vi "PicoScope4000aProbeSettings.vi"(0 "handle in":i16, 1 "Device Info":T3={"Driver Version"="", "USB Version"="", "Hardware"="", "Variant"="", "Batch and Serial"="", "Cal Date"="", "Kernel Version"="", "Digital HW Version"="", "Analogue HW Version"="", "Firmware 1"="", "Firmware 2"="", "Num. channels"=4}, 4 "Probe Input Array":T5(array[cluster])=[{"probeNumber"=0, FALSE, "channel"=-1, "enabled"=0, "probeName"=0, "requiresPower"=0, "isPowered"=0, "probeOff"=0, "rangeFirst"=0, "rangeLast"=0, "rangeCurrent"=0, "couplingFirst"=0, "couplingLast"=0, "couplingCurrent"=0, "filterFlags"=0, "filterCurrent"=0, "defaultFilter"=0}, {"probeNumber"=0, FALSE, "channel"=-1, "enabled"=0, "probeName"=0, "requiresPower"=0, "isPowered"=0, "probeOff"=0, "rangeFirst"=0, "rangeLast"=0, "rangeCurrent"=0, "couplingFirst"=0, "couplingLast"=0, "couplingCurrent"=0, "filterFlags"=0, "filterCurrent"=0, "defaultFilter"=0}, {"probeNumber"=0, FALSE, "channel"=-1, "enabled"=0, "probeName"=0, "requiresPower"=0, "isPowered"=0, "probeOff"=0, "rangeFirst"=0, "rangeLast"=0, "rangeCurrent"=0, "couplingFirst"=0, "couplingLast"=0, "couplingCurrent"=0, "filterFlags"=0, "filterCurrent"=0, "defaultFilter"=0}, {"probeNumber"=0, FALSE, "channel"=-1, "enabled"=0, "probeName"=0, "requiresPower"=0, "isPowered"=0, "probeOff"=0, "rangeFirst"=0, "rangeLast"=0, "rangeCurrent"=0, "couplingFirst"=0, "couplingLast"=0, "couplingCurrent"=0, "filterFlags"=0, "filterCurrent"=0, "defaultFilter"=0}], 5 "error in (no error)":errorcluster, 6 "Channel A Settings":T4={"Enabled"=FALSE, "Coupling"=1, "Range"=0, "Analogue Offset"=0.0, "Bandwidth Limit"=0} {"Range" items=["10mV"=0, "20mV"=1, "50mV"=2, "100mV"=3, "200mV"=4, "500mV"=5, "1V"=6, "2V"=7, "5V"=8, "10V"=9, "20V"=10, "50V"=11, "100V"=12, "200V"=13, "1KV_2_5V"=6003, "1KV_5V"=6004, "1KV_12_5V"=6005, "1KV_25V"=6006, "1KV_50V"=6007, "1KV_125V"=6008, "1KV_250V"=6009, "1KV_500V"=6010, "1KV_1000V"=6011, "CURRENT_CLAMP_200A_2kA_1A"=4000, "CURRENT_CLAMP_200A_2kA_2A"=4001, "CURRENT_CLAMP_200A_2kA_5A"=4002, "CURRENT_CLAMP_200A_2kA_10A"=4003, "CURRENT_CLAMP_200A_2kA_20A"=4004, "CURRENT_CLAMP_200A_2kA_50A"=4005, "CURRENT_CLAMP_200A_2kA_100A"=4006, "CURRENT_CLAMP_200A_2kA_200A"=4007, "CURRENT_CLAMP_200A_2kA_500A"=4008, "CURRENT_CLAMP_200A_2kA_1000A"=4009, "CURRENT_CLAMP_200A_2kA_2000A"=4010, "CURRENT_CLAMP_40A_100mA"=5000, "CURRENT_CLAMP_40A_200mA"=5001, "CURRENT_CLAMP_40A_500mA"=5002, "CURRENT_CLAMP_40A_1A"=5003, "CURRENT_CLAMP_40A_2A"=5004, "CURRENT_CLAMP_40A_5A"=5005, "CURRENT_CLAMP_40A_10A"=5006, "CURRENT_CLAMP_40A_20A"=5007, "CURRENT_CLAMP_40A_40A"=5008, "CURRENT_CLAMP_2000ARMS_10A"=6500, "CURRENT_CLAMP_2000ARMS_20A"=6501, "CURRENT_CLAMP_2000ARMS_50A"=6502, "CURRENT_CLAMP_2000ARMS_100A"=6503, "CURRENT_CLAMP_2000ARMS_200A"=6504, "CURRENT_CLAMP_2000ARMS_500A"=6505, "CURRENT_CLAMP_2000ARMS_1000A"=6506, "CURRENT_CLAMP_2000ARMS_2000A"=6507, "CURRENT_CLAMP_2000ARMS_5000A"=6508, "x10_Probe_100mV"=32, "x10_Probe_200mV"=33, "x10_Probe_500mV"=34, "x10_Probe_1V"=35, "x10_Probe_2V"=36, "x10_Probe_5V"=37, "x10_Probe_10V"=38, "x10_Probe_20V"=39, "x10_Probe_50V"=40, "x10_Probe_100V"=41, "x10_Probe_200V"=42, "x10_Probe_500V"=43, "CURRENT_CLAMP_60A_2A"=10500, "CURRENT_CLAMP_60A_5A"=10501, "CURRENT_CLAMP_60A_10A"=10502, "CURRENT_CLAMP_60A_20A"=10503, "CURRENT_CLAMP_60A_50A"=10504, "CURRENT_CLAMP_60A_60A"=10505, "CURRENT_CLAMP_60A_V2_0_5A"=10600, "CURRENT_CLAMP_60A_V2_1A"=10601, "CURRENT_CLAMP_60A_V2_2A"=10602, "CURRENT_CLAMP_60A_V2_5A"=10603, "CURRENT_CLAMP_60A_V2_10A"=10604, "CURRENT_CLAMP_60A_V2_20A"=10605, "CURRENT_CLAMP_60A_V2_50A"=10606, "CURRENT_CLAMP_60A_V2_60A"=10607, "RESISTANCE_LEAD_NEG5_TO_20OHM"=7000, "RESISTANCE_LEAD_NEG50_TO_200OHM"=7001, "RESISTANCE_LEAD_NEG500_TO_2KOHM"=7002, "RESISTANCE_LEAD_NEG5K_TO_20KOHM"=7003, "RESISTANCE_LEAD_NEG50K_TO_LEAD_200KOHM"=7004, "RESISTANCE_LEAD_NEG500K_TO_LEAD_2MOHM"=7005, "RESISTANCE_LEAD_DIODE_TEST"=7006, "HT_NEG3_TO_5KV"=8950, "HT_NEG3_TO_10KV"=8951, "HT_NEG5_TO_20KV"=8952, "HT_NEG5_TO_50KV"=8953, "HT_NEG5_TO_100KV"=8954, "HT_NEG3_TO_5KV_INVERTED"=8955, "HT_NEG3_TO_10KV_INVERTED"=8956, "HT_NEG5_TO_20KV_INVERTED"=8957, "HT_NEG5_TO_50KV_INVERTED"=8958, "HT_NEG5_TO_100KV_INVERTED"=8959, "TEMPERATURE_NEG50_TO_150DEGC"=9000, "PRESSURE_SENSOR_-100k-150k_PASCALS"=9100, "PRESSURE_SENSOR_-100k_TO_400k_PASCALS"=9101, "PRESSURE_SENSOR_-200k_TO_800k_PASCALS"=9102, "PRESSURE_SENSOR_-400k_TO_1600k_PASCALS"=9103, "PRESSURE_SENSOR_-400k_TO_3400k_PASCALS"=9104, "PRESSURE_SENSOR_-150k_TO_1350k_PASCALS"=9105, "PICO_CONNECT_PROBE_OFF"=1024]; "Bandwidth Limit" items=["Full", "20kHz", "100kHz", "1MHz"]; "Coupling" items=["AC", "DC"]}, 8 "Channel B Settings":T4={"Enabled"=FALSE, "Coupling"=1, "Range"=0, "Analogue Offset"=0.0, "Bandwidth Limit"=0} {"Range" items=["10mV"=0, "20mV"=1, "50mV"=2, "100mV"=3, "200mV"=4, "500mV"=5, "1V"=6, "2V"=7, "5V"=8, "10V"=9, "20V"=10, "50V"=11, "100V"=12, "200V"=13, "1KV_2_5V"=6003, "1KV_5V"=6004, "1KV_12_5V"=6005, "1KV_25V"=6006, "1KV_50V"=6007, "1KV_125V"=6008, "1KV_250V"=6009, "1KV_500V"=6010, "1KV_1000V"=6011, "CURRENT_CLAMP_200A_2kA_1A"=4000, "CURRENT_CLAMP_200A_2kA_2A"=4001, "CURRENT_CLAMP_200A_2kA_5A"=4002, "CURRENT_CLAMP_200A_2kA_10A"=4003, "CURRENT_CLAMP_200A_2kA_20A"=4004, "CURRENT_CLAMP_200A_2kA_50A"=4005, "CURRENT_CLAMP_200A_2kA_100A"=4006, "CURRENT_CLAMP_200A_2kA_200A"=4007, "CURRENT_CLAMP_200A_2kA_500A"=4008, "CURRENT_CLAMP_200A_2kA_1000A"=4009, "CURRENT_CLAMP_200A_2kA_2000A"=4010, "CURRENT_CLAMP_40A_100mA"=5000, "CURRENT_CLAMP_40A_200mA"=5001, "CURRENT_CLAMP_40A_500mA"=5002, "CURRENT_CLAMP_40A_1A"=5003, "CURRENT_CLAMP_40A_2A"=5004, "CURRENT_CLAMP_40A_5A"=5005, "CURRENT_CLAMP_40A_10A"=5006, "CURRENT_CLAMP_40A_20A"=5007, "CURRENT_CLAMP_40A_40A"=5008, "CURRENT_CLAMP_2000ARMS_10A"=6500, "CURRENT_CLAMP_2000ARMS_20A"=6501, "CURRENT_CLAMP_2000ARMS_50A"=6502, "CURRENT_CLAMP_2000ARMS_100A"=6503, "CURRENT_CLAMP_2000ARMS_200A"=6504, "CURRENT_CLAMP_2000ARMS_500A"=6505, "CURRENT_CLAMP_2000ARMS_1000A"=6506, "CURRENT_CLAMP_2000ARMS_2000A"=6507, "CURRENT_CLAMP_2000ARMS_5000A"=6508, "x10_Probe_100mV"=32, "x10_Probe_200mV"=33, "x10_Probe_500mV"=34, "x10_Probe_1V"=35, "x10_Probe_2V"=36, "x10_Probe_5V"=37, "x10_Probe_10V"=38, "x10_Probe_20V"=39, "x10_Probe_50V"=40, "x10_Probe_100V"=41, "x10_Probe_200V"=42, "x10_Probe_500V"=43, "CURRENT_CLAMP_60A_2A"=10500, "CURRENT_CLAMP_60A_5A"=10501, "CURRENT_CLAMP_60A_10A"=10502, "CURRENT_CLAMP_60A_20A"=10503, "CURRENT_CLAMP_60A_50A"=10504, "CURRENT_CLAMP_60A_60A"=10505, "CURRENT_CLAMP_60A_V2_0_5A"=10600, "CURRENT_CLAMP_60A_V2_1A"=10601, "CURRENT_CLAMP_60A_V2_2A"=10602, "CURRENT_CLAMP_60A_V2_5A"=10603, "CURRENT_CLAMP_60A_V2_10A"=10604, "CURRENT_CLAMP_60A_V2_20A"=10605, "CURRENT_CLAMP_60A_V2_50A"=10606, "CURRENT_CLAMP_60A_V2_60A"=10607, "RESISTANCE_LEAD_NEG5_TO_20OHM"=7000, "RESISTANCE_LEAD_NEG50_TO_200OHM"=7001, "RESISTANCE_LEAD_NEG500_TO_2KOHM"=7002, "RESISTANCE_LEAD_NEG5K_TO_20KOHM"=7003, "RESISTANCE_LEAD_NEG50K_TO_LEAD_200KOHM"=7004, "RESISTANCE_LEAD_NEG500K_TO_LEAD_2MOHM"=7005, "RESISTANCE_LEAD_DIODE_TEST"=7006, "HT_NEG3_TO_5KV"=8950, "HT_NEG3_TO_10KV"=8951, "HT_NEG5_TO_20KV"=8952, "HT_NEG5_TO_50KV"=8953, "HT_NEG5_TO_100KV"=8954, "HT_NEG3_TO_5KV_INVERTED"=8955, "HT_NEG3_TO_10KV_INVERTED"=8956, "HT_NEG5_TO_20KV_INVERTED"=8957, "HT_NEG5_TO_50KV_INVERTED"=8958, "HT_NEG5_TO_100KV_INVERTED"=8959, "TEMPERATURE_NEG50_TO_150DEGC"=9000, "PRESSURE_SENSOR_-100k-150k_PASCALS"=9100, "PRESSURE_SENSOR_-100k_TO_400k_PASCALS"=9101, "PRESSURE_SENSOR_-200k_TO_800k_PASCALS"=9102, "PRESSURE_SENSOR_-400k_TO_1600k_PASCALS"=9103, "PRESSURE_SENSOR_-400k_TO_3400k_PASCALS"=9104, "PRESSURE_SENSOR_-150k_TO_1350k_PASCALS"=9105, "PICO_CONNECT_PROBE_OFF"=1024]; "Bandwidth Limit" items=["Full", "20kHz", "100kHz", "1MHz"]; "Coupling" items=["AC", "DC"]}, 10 "Channel C Settings":T4={"Enabled"=FALSE, "Coupling"=1, "Range"=0, "Analogue Offset"=0.0, "Bandwidth Limit"=0} {"Range" items=["10mV"=0, "20mV"=1, "50mV"=2, "100mV"=3, "200mV"=4, "500mV"=5, "1V"=6, "2V"=7, "5V"=8, "10V"=9, "20V"=10, "50V"=11, "100V"=12, "200V"=13, "1KV_2_5V"=6003, "1KV_5V"=6004, "1KV_12_5V"=6005, "1KV_25V"=6006, "1KV_50V"=6007, "1KV_125V"=6008, "1KV_250V"=6009, "1KV_500V"=6010, "1KV_1000V"=6011, "CURRENT_CLAMP_200A_2kA_1A"=4000, "CURRENT_CLAMP_200A_2kA_2A"=4001, "CURRENT_CLAMP_200A_2kA_5A"=4002, "CURRENT_CLAMP_200A_2kA_10A"=4003, "CURRENT_CLAMP_200A_2kA_20A"=4004, "CURRENT_CLAMP_200A_2kA_50A"=4005, "CURRENT_CLAMP_200A_2kA_100A"=4006, "CURRENT_CLAMP_200A_2kA_200A"=4007, "CURRENT_CLAMP_200A_2kA_500A"=4008, "CURRENT_CLAMP_200A_2kA_1000A"=4009, "CURRENT_CLAMP_200A_2kA_2000A"=4010, "CURRENT_CLAMP_40A_100mA"=5000, "CURRENT_CLAMP_40A_200mA"=5001, "CURRENT_CLAMP_40A_500mA"=5002, "CURRENT_CLAMP_40A_1A"=5003, "CURRENT_CLAMP_40A_2A"=5004, "CURRENT_CLAMP_40A_5A"=5005, "CURRENT_CLAMP_40A_10A"=5006, "CURRENT_CLAMP_40A_20A"=5007, "CURRENT_CLAMP_40A_40A"=5008, "CURRENT_CLAMP_2000ARMS_10A"=6500, "CURRENT_CLAMP_2000ARMS_20A"=6501, "CURRENT_CLAMP_2000ARMS_50A"=6502, "CURRENT_CLAMP_2000ARMS_100A"=6503, "CURRENT_CLAMP_2000ARMS_200A"=6504, "CURRENT_CLAMP_2000ARMS_500A"=6505, "CURRENT_CLAMP_2000ARMS_1000A"=6506, "CURRENT_CLAMP_2000ARMS_2000A"=6507, "CURRENT_CLAMP_2000ARMS_5000A"=6508, "x10_Probe_100mV"=32, "x10_Probe_200mV"=33, "x10_Probe_500mV"=34, "x10_Probe_1V"=35, "x10_Probe_2V"=36, "x10_Probe_5V"=37, "x10_Probe_10V"=38, "x10_Probe_20V"=39, "x10_Probe_50V"=40, "x10_Probe_100V"=41, "x10_Probe_200V"=42, "x10_Probe_500V"=43, "CURRENT_CLAMP_60A_2A"=10500, "CURRENT_CLAMP_60A_5A"=10501, "CURRENT_CLAMP_60A_10A"=10502, "CURRENT_CLAMP_60A_20A"=10503, "CURRENT_CLAMP_60A_50A"=10504, "CURRENT_CLAMP_60A_60A"=10505, "CURRENT_CLAMP_60A_V2_0_5A"=10600, "CURRENT_CLAMP_60A_V2_1A"=10601, "CURRENT_CLAMP_60A_V2_2A"=10602, "CURRENT_CLAMP_60A_V2_5A"=10603, "CURRENT_CLAMP_60A_V2_10A"=10604, "CURRENT_CLAMP_60A_V2_20A"=10605, "CURRENT_CLAMP_60A_V2_50A"=10606, "CURRENT_CLAMP_60A_V2_60A"=10607, "RESISTANCE_LEAD_NEG5_TO_20OHM"=7000, "RESISTANCE_LEAD_NEG50_TO_200OHM"=7001, "RESISTANCE_LEAD_NEG500_TO_2KOHM"=7002, "RESISTANCE_LEAD_NEG5K_TO_20KOHM"=7003, "RESISTANCE_LEAD_NEG50K_TO_LEAD_200KOHM"=7004, "RESISTANCE_LEAD_NEG500K_TO_LEAD_2MOHM"=7005, "RESISTANCE_LEAD_DIODE_TEST"=7006, "HT_NEG3_TO_5KV"=8950, "HT_NEG3_TO_10KV"=8951, "HT_NEG5_TO_20KV"=8952, "HT_NEG5_TO_50KV"=8953, "HT_NEG5_TO_100KV"=8954, "HT_NEG3_TO_5KV_INVERTED"=8955, "HT_NEG3_TO_10KV_INVERTED"=8956, "HT_NEG5_TO_20KV_INVERTED"=8957, "HT_NEG5_TO_50KV_INVERTED"=8958, "HT_NEG5_TO_100KV_INVERTED"=8959, "TEMPERATURE_NEG50_TO_150DEGC"=9000, "PRESSURE_SENSOR_-100k-150k_PASCALS"=9100, "PRESSURE_SENSOR_-100k_TO_400k_PASCALS"=9101, "PRESSURE_SENSOR_-200k_TO_800k_PASCALS"=9102, "PRESSURE_SENSOR_-400k_TO_1600k_PASCALS"=9103, "PRESSURE_SENSOR_-400k_TO_3400k_PASCALS"=9104, "PRESSURE_SENSOR_-150k_TO_1350k_PASCALS"=9105, "PICO_CONNECT_PROBE_OFF"=1024]; "Bandwidth Limit" items=["Full", "20kHz", "100kHz", "1MHz"]; "Coupling" items=["AC", "DC"]}, 12 "Channel D Settings":T4={"Enabled"=FALSE, "Coupling"=1, "Range"=0, "Analogue Offset"=0.0, "Bandwidth Limit"=0} {"Range" items=["10mV"=0, "20mV"=1, "50mV"=2, "100mV"=3, "200mV"=4, "500mV"=5, "1V"=6, "2V"=7, "5V"=8, "10V"=9, "20V"=10, "50V"=11, "100V"=12, "200V"=13, "1KV_2_5V"=6003, "1KV_5V"=6004, "1KV_12_5V"=6005, "1KV_25V"=6006, "1KV_50V"=6007, "1KV_125V"=6008, "1KV_250V"=6009, "1KV_500V"=6010, "1KV_1000V"=6011, "CURRENT_CLAMP_200A_2kA_1A"=4000, "CURRENT_CLAMP_200A_2kA_2A"=4001, "CURRENT_CLAMP_200A_2kA_5A"=4002, "CURRENT_CLAMP_200A_2kA_10A"=4003, "CURRENT_CLAMP_200A_2kA_20A"=4004, "CURRENT_CLAMP_200A_2kA_50A"=4005, "CURRENT_CLAMP_200A_2kA_100A"=4006, "CURRENT_CLAMP_200A_2kA_200A"=4007, "CURRENT_CLAMP_200A_2kA_500A"=4008, "CURRENT_CLAMP_200A_2kA_1000A"=4009, "CURRENT_CLAMP_200A_2kA_2000A"=4010, "CURRENT_CLAMP_40A_100mA"=5000, "CURRENT_CLAMP_40A_200mA"=5001, "CURRENT_CLAMP_40A_500mA"=5002, "CURRENT_CLAMP_40A_1A"=5003, "CURRENT_CLAMP_40A_2A"=5004, "CURRENT_CLAMP_40A_5A"=5005, "CURRENT_CLAMP_40A_10A"=5006, "CURRENT_CLAMP_40A_20A"=5007, "CURRENT_CLAMP_40A_40A"=5008, "CURRENT_CLAMP_2000ARMS_10A"=6500, "CURRENT_CLAMP_2000ARMS_20A"=6501, "CURRENT_CLAMP_2000ARMS_50A"=6502, "CURRENT_CLAMP_2000ARMS_100A"=6503, "CURRENT_CLAMP_2000ARMS_200A"=6504, "CURRENT_CLAMP_2000ARMS_500A"=6505, "CURRENT_CLAMP_2000ARMS_1000A"=6506, "CURRENT_CLAMP_2000ARMS_2000A"=6507, "CURRENT_CLAMP_2000ARMS_5000A"=6508, "x10_Probe_100mV"=32, "x10_Probe_200mV"=33, "x10_Probe_500mV"=34, "x10_Probe_1V"=35, "x10_Probe_2V"=36, "x10_Probe_5V"=37, "x10_Probe_10V"=38, "x10_Probe_20V"=39, "x10_Probe_50V"=40, "x10_Probe_100V"=41, "x10_Probe_200V"=42, "x10_Probe_500V"=43, "CURRENT_CLAMP_60A_2A"=10500, "CURRENT_CLAMP_60A_5A"=10501, "CURRENT_CLAMP_60A_10A"=10502, "CURRENT_CLAMP_60A_20A"=10503, "CURRENT_CLAMP_60A_50A"=10504, "CURRENT_CLAMP_60A_60A"=10505, "CURRENT_CLAMP_60A_V2_0_5A"=10600, "CURRENT_CLAMP_60A_V2_1A"=10601, "CURRENT_CLAMP_60A_V2_2A"=10602, "CURRENT_CLAMP_60A_V2_5A"=10603, "CURRENT_CLAMP_60A_V2_10A"=10604, "CURRENT_CLAMP_60A_V2_20A"=10605, "CURRENT_CLAMP_60A_V2_50A"=10606, "CURRENT_CLAMP_60A_V2_60A"=10607, "RESISTANCE_LEAD_NEG5_TO_20OHM"=7000, "RESISTANCE_LEAD_NEG50_TO_200OHM"=7001, "RESISTANCE_LEAD_NEG500_TO_2KOHM"=7002, "RESISTANCE_LEAD_NEG5K_TO_20KOHM"=7003, "RESISTANCE_LEAD_NEG50K_TO_LEAD_200KOHM"=7004, "RESISTANCE_LEAD_NEG500K_TO_LEAD_2MOHM"=7005, "RESISTANCE_LEAD_DIODE_TEST"=7006, "HT_NEG3_TO_5KV"=8950, "HT_NEG3_TO_10KV"=8951, "HT_NEG5_TO_20KV"=8952, "HT_NEG5_TO_50KV"=8953, "HT_NEG5_TO_100KV"=8954, "HT_NEG3_TO_5KV_INVERTED"=8955, "HT_NEG3_TO_10KV_INVERTED"=8956, "HT_NEG5_TO_20KV_INVERTED"=8957, "HT_NEG5_TO_50KV_INVERTED"=8958, "HT_NEG5_TO_100KV_INVERTED"=8959, "TEMPERATURE_NEG50_TO_150DEGC"=9000, "PRESSURE_SENSOR_-100k-150k_PASCALS"=9100, "PRESSURE_SENSOR_-100k_TO_400k_PASCALS"=9101, "PRESSURE_SENSOR_-200k_TO_800k_PASCALS"=9102, "PRESSURE_SENSOR_-400k_TO_1600k_PASCALS"=9103, "PRESSURE_SENSOR_-400k_TO_3400k_PASCALS"=9104, "PRESSURE_SENSOR_-150k_TO_1350k_PASCALS"=9105, "PICO_CONNECT_PROBE_OFF"=1024]; "Bandwidth Limit" items=["Full", "20kHz", "100kHz", "1MHz"]; "Coupling" items=["AC", "DC"]}) -> (7 "ChA":T2={"Probe Info"={"Ch Min Limit"=0.0, "Ch Max Limit"=0.0, "Probe Name"=0}, "Channel A Settings "={"Enabled"=FALSE, "Coupling"=1, "Range"=0, "Analogue Offset"=0.0, "Bandwidth Limit"=0}} {"Channel A Settings"."Bandwidth Limit" items=["Full", "20kHz", "100kHz", "1MHz"]; "Channel A Settings"."Range" items=["10 mV", "20 mV", "50 mV", "100 mV", "200 mV", "500 mV", "1 V", "2 V", "5 V", "10 V", "20 V", "50 V ", "100 V"]; "Channel A Settings"."Coupling" items=["AC", "DC"]}, 9 "ChB":T2={"Probe Info"={"Ch Min Limit"=0.0, "Ch Max Limit"=0.0, "Probe Name"=0}, "Channel A Settings "={"Enabled"=FALSE, "Coupling"=1, "Range"=0, "Analogue Offset"=0.0, "Bandwidth Limit"=0}} {"Channel A Settings"."Bandwidth Limit" items=["Full", "20kHz", "100kHz", "1MHz"]; "Channel A Settings"."Range" items=["10 mV", "20 mV", "50 mV", "100 mV", "200 mV", "500 mV", "1 V", "2 V", "5 V", "10 V", "20 V", "50 V ", "100 V"]; "Channel A Settings"."Coupling" items=["AC", "DC"]}, 11 "ChC":T2={"Probe Info"={"Ch Min Limit"=0.0, "Ch Max Limit"=0.0, "Probe Name"=0}, "Channel A Settings "={"Enabled"=FALSE, "Coupling"=1, "Range"=0, "Analogue Offset"=0.0, "Bandwidth Limit"=0}} {"Channel A Settings"."Bandwidth Limit" items=["Full", "20kHz", "100kHz", "1MHz"]; "Channel A Settings"."Range" items=["10 mV", "20 mV", "50 mV", "100 mV", "200 mV", "500 mV", "1 V", "2 V", "5 V", "10 V", "20 V", "50 V ", "100 V"]; "Channel A Settings"."Coupling" items=["AC", "DC"]}, 13 "ChD":T2={"Probe Info"={"Ch Min Limit"=0.0, "Ch Max Limit"=0.0, "Probe Name"=0}, "Channel A Settings "={"Enabled"=FALSE, "Coupling"=1, "Range"=0, "Analogue Offset"=0.0, "Bandwidth Limit"=0}} {"Channel A Settings"."Bandwidth Limit" items=["Full", "20kHz", "100kHz", "1MHz"]; "Channel A Settings"."Range" items=["10 mV", "20 mV", "50 mV", "100 mV", "200 mV", "500 mV", "1 V", "2 V", "5 V", "10 V", "20 V", "50 V ", "100 V"]; "Channel A Settings"."Coupling" items=["AC", "DC"]}, 14 "handle out":i16, 19 "error out":errorcluster)   [LabVIEW 2010]
uses:
  PicoScope4000aAnalogChannelSettings.ctl
  PicoScope4000aAnalogChannelSettings_PicoConnect.ctl
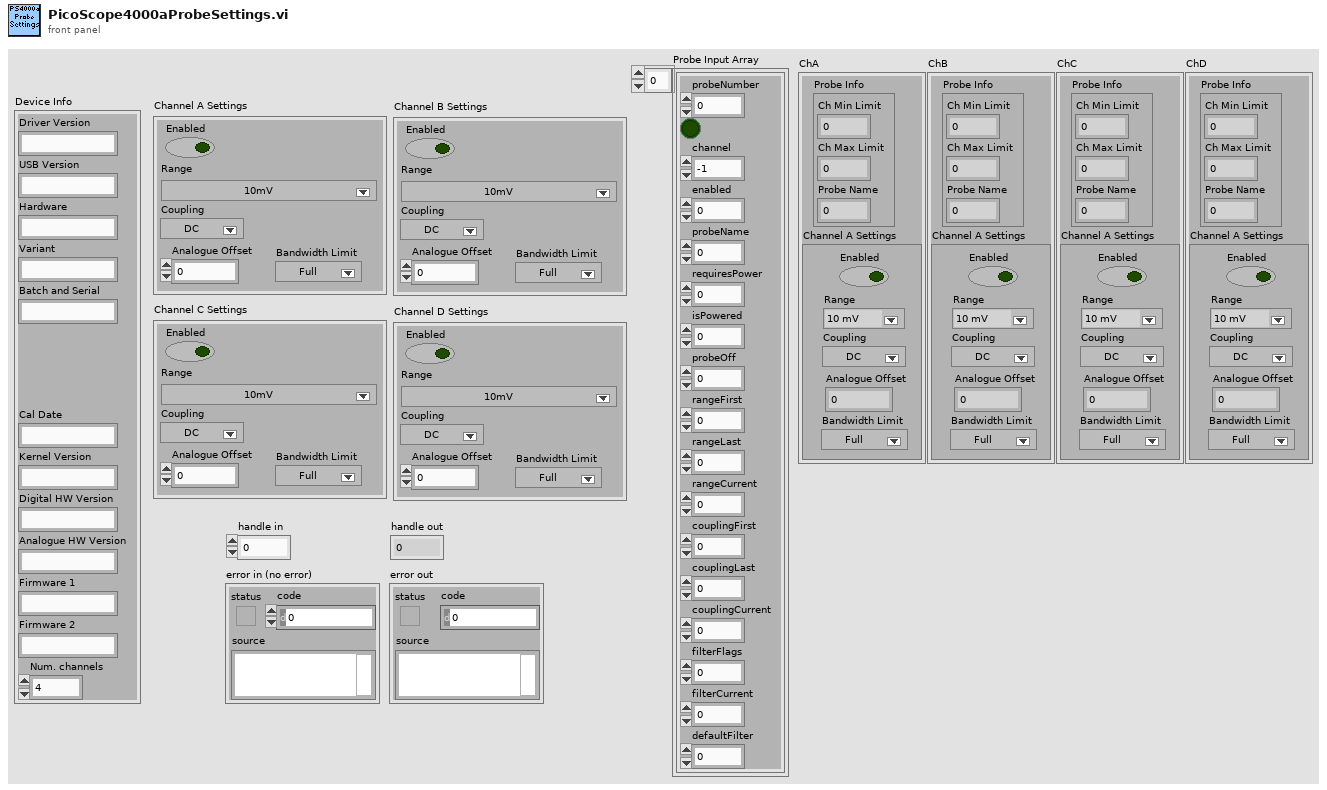
[diagram p1: front panel]
types:
  T1 = typedef "PicoScope4000aAnalogChannelSettings.ctl" = cluster{"Enabled":bool, "Coupling":i16, "Range":u32, "Analogue Offset":sgl, "Bandwidth Limit":u32}
  T2 = cluster{"Probe Info":cluster{"Ch Min Limit":dbl, "Ch Max Limit":dbl, "Probe Name":i32}, "Channel A Settings ":T1}
  T3 = cluster{"Driver Version":string, "USB Version":string, "Hardware":string, "Variant":string, "Batch and Serial":string, "Cal Date":string, "Kernel Version":string, "Digital HW Version":string, "Analogue HW Version":string, "Firmware 1":string, "Firmware 2":string, "Num. channels":i16}
  T4 = typedef "PicoScope4000aAnalogChannelSettings_PicoConnect.ctl" = cluster{"Enabled":bool, "Coupling":i16, "Range":u32, "Analogue Offset":sgl, "Bandwidth Limit":u32}
  T5 = cluster{"probeNumber":i32, bool, "channel":i32, "enabled":i16, "probeName":i32, "requiresPower":i8, "isPowered":i8, "probeOff":i32, "rangeFirst":i32, "rangeLast":i32, "rangeCurrent":i32, "couplingFirst":i32, "couplingLast":i32, "couplingCurrent":i32, "filterFlags":i32, "filterCurrent":i32, "defaultFilter":i32}[]
  T6 = cluster{"Ch Min Limit":dbl, "Ch Max Limit":dbl, "Probe Name":i32}
  T7 = cluster{"probeNumber":i32, bool, "channel":i32, "enabled":i16, "probeName":i32, "requiresPower":i8, "isPowered":i8, "probeOff":i32, "rangeFirst":i32, "rangeLast":i32, "rangeCurrent":i32, "couplingFirst":i32, "couplingLast":i32, "couplingCurrent":i32, "filterFlags":i32, "filterCurrent":i32, "defaultFilter":i32}
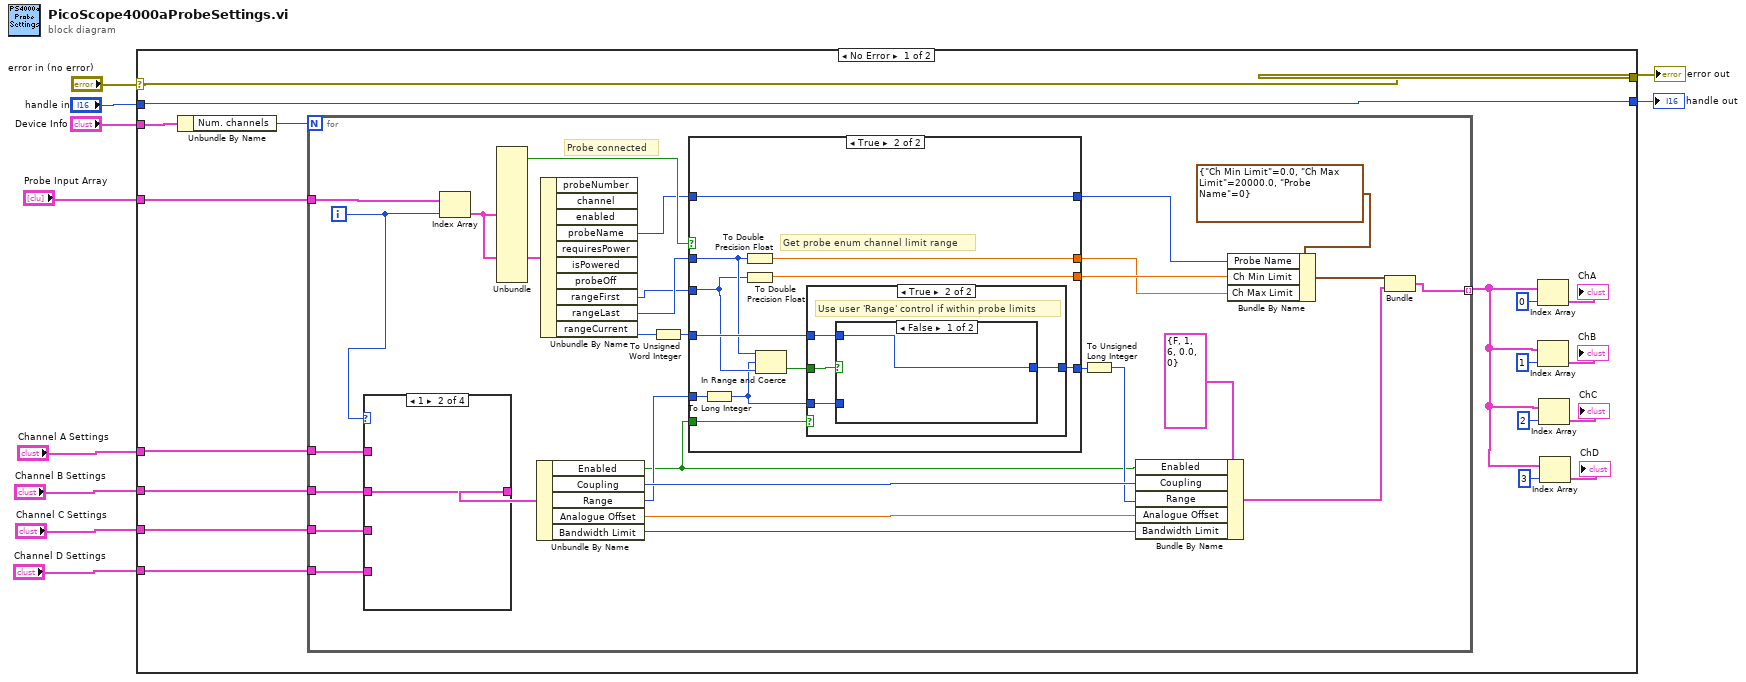
[diagram p0: block diagram]
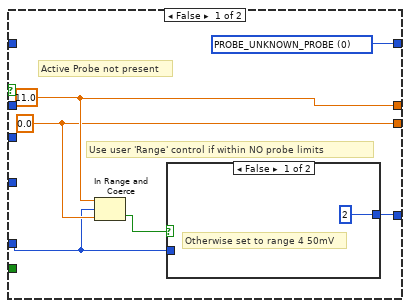
[diagram p5: hidden frame]
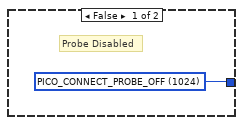
[diagram p7: hidden frame]
diagram:
  n1 = case shown="No Error" "error in (no error)" {
    selector: "error in (no error)" -> [w25 w89]
    tunnel: "handle in" -> [w27 w88]
    tunnel: [w27 w88] -> w10
    tunnel: [w25 w89] -> w9
    tunnel: "Device Info" -> [w16 _]
    tunnel: "Channel A Settings" -> [w28 _]
    tunnel: "Probe Input Array" -> [w26 _]
    tunnel: "Channel B Settings" -> [w24 _]
    tunnel: "Channel C Settings" -> [w23 _]
    tunnel: "Channel D Settings" -> [w22 _]
    frame No Error {
      n2 = Unbundle By Name(w16) -> ("Num. channels"=w15:i16)
      n3 = for {
        N: w15 -> [_]
        tunnel: w28 -> [w38]
        tunnel: w26 -> [w53]
        tunnel: w24 -> [w39]
        tunnel: w23 -> [w37]
        tunnel: w22 -> [w36]
        tunnel: [w35] -> w17 mode=indexing
        i -> [w41]
        # "Probe connected"
        n4 = case shown="1" w41 {
          tunnel: [w58 w59 w60 w61] -> w40
          tunnel: w39 -> [_ w59 _ _]
          tunnel: w38 -> [w58 _ _ _]
          tunnel: w37 -> [_ _ w60 _]
          tunnel: w36 -> [_ _ _ w61]
          frame 0, Default {
          }
          frame 1 {
          }
          frame 2 {
          }
          frame 3 {
          }
        }
        n5 = Index Array(array=w53, index=w41) -> (element=w52:T7)
        n6 = Unbundle(w52) -> (w51:bool)  [unwired: 16 out]
        n7 = Unbundle By Name(w40) -> ("Enabled"=w31:bool, "Coupling"=w57:i16, "Range"=w48:u32, "Analogue Offset"=w56:sgl, "Bandwidth Limit"=w30:u32)
        n8 = Unbundle By Name(w52) -> ("probeName"=w32:i32, "rangeFirst"=w54:i32, "rangeLast"=w55:i32, "rangeCurrent"=w50:i32)  [unwired: 6 out]
        n9 = To Unsigned Word Integer(number=w50) -> (unsigned 16bit integer=w47:u16)
        n10 = case shown="True" w51 {
          tunnel: w48 -> [w64 w78]
          tunnel: [w66 w79] -> w42
          tunnel: [w65 w80] -> w43
          tunnel: w55 -> [_ w75]
          tunnel: w54 -> [_ w74]
          tunnel: w47 -> [_ w76]
          tunnel: [w63 w72] -> w46
          tunnel: [w62 w71] -> w33
          tunnel: w32 -> [_ w71]
          tunnel: w31 -> [_ w70]
          frame False {
            w62 = 0 items=["PROBE_D9_BNC"=4000, "PROBE_D9_2X_BNC"=4001, "PROBE_DIFFERENTIAL"=4002, "PROBE_CURRENT_CLAMP_200_2KA"=4003, "CONNECT_PROBE_CURRENT_CLAMP_40A"=4004, "CONNECT_PROBE_CAT3_HV_1KV"=4005, "CONNECT_PROBE_CURRENT_CLAMP_2000ARMS"=4006, "PROBE_UNKNOWN_PROBE"=0] ("Probe Name")
            w65 = 0.0 ("Data Entry Limits:Minimum")
            w66 = 11.0 ("Data Entry Limits:Maximum")
            # "Use user 'Range' control if within NO probe limits"
            # "Active Probe not present"
            n11 = In Range and Coerce(upper limit=w66, x=w64, lower limit=w65) -> (In Range?=w67:bool)  [unwired: 1 out]
            n12 = case shown="False" w67 {
              tunnel: [u16 2 ("Range") w69] -> w63
              tunnel: w64 -> [_ w69]
              frame False {
                # "Otherwise set to range 4 50mV"
              }
              frame True {
              }
            }
          }
          frame True {
            # "Get probe enum channel limit range"
            n13 = To Long Integer(number=w78) -> (32bit integer=w73:i32)
            n14 = To Double Precision Float(number=w75) -> (double precision float=w79:dbl)
            n15 = To Double Precision Float(number=w74) -> (double precision float=w80:dbl)
            n16 = In Range and Coerce(upper limit=w75, x=w73, lower limit=w74) -> (In Range?=w77:bool)  [unwired: 1 out]
            n17 = case shown="True" w70 {
              tunnel: w77 -> [_ w85]
              tunnel: w76 -> [_ w84]
              tunnel: w73 -> [_ w83]
              tunnel: [w81 w82] -> w72
              frame False {
                w81 = u32 1024 items=["10mV"=0, "20mV"=1, "50mV"=2, "100mV"=3, "200mV"=4, "500mV"=5, "1V"=6, "2V"=7, "5V"=8, "10V"=9, "20V"=10, "50V"=11, "100V"=12, "200V"=13, "1KV_2_5V"=6003, "1KV_5V"=6004, "1KV_12_5V"=6005, "1KV_25V"=6006, "1KV_50V"=6007, "1KV_125V"=6008, "1KV_250V"=6009, "1KV_500V"=6010, "1KV_1000V"=6011, "CURRENT_CLAMP_200A_2kA_1A"=4000, "CURRENT_CLAMP_200A_2kA_2A"=4001, "CURRENT_CLAMP_200A_2kA_5A"=4002, "CURRENT_CLAMP_200A_2kA_10A"=4003, "CURRENT_CLAMP_200A_2kA_20A"=4004, "CURRENT_CLAMP_200A_2kA_50A"=4005, "CURRENT_CLAMP_200A_2kA_100A"=4006, "CURRENT_CLAMP_200A_2kA_200A"=4007, "CURRENT_CLAMP_200A_2kA_500A"=4008, "CURRENT_CLAMP_200A_2kA_1000A"=4009, "CURRENT_CLAMP_200A_2kA_2000A"=4010, "CURRENT_CLAMP_40A_100mA"=5000, "CURRENT_CLAMP_40A_200mA"=5001, "CURRENT_CLAMP_40A_500mA"=5002, "CURRENT_CLAMP_40A_1A"=5003, "CURRENT_CLAMP_40A_2A"=5004, "CURRENT_CLAMP_40A_5A"=5005, "CURRENT_CLAMP_40A_10A"=5006, "CURRENT_CLAMP_40A_20A"=5007, "CURRENT_CLAMP_40A_40A"=5008, "CURRENT_CLAMP_2000ARMS_10A"=6500, "CURRENT_CLAMP_2000ARMS_20A"=6501, "CURRENT_CLAMP_2000ARMS_50A"=6502, "CURRENT_CLAMP_2000ARMS_100A"=6503, "CURRENT_CLAMP_2000ARMS_200A"=6504, "CURRENT_CLAMP_2000ARMS_500A"=6505, "CURRENT_CLAMP_2000ARMS_1000A"=6506, "CURRENT_CLAMP_2000ARMS_2000A"=6507, "CURRENT_CLAMP_2000ARMS_5000A"=6508, "x10_Probe_100mV"=32, "x10_Probe_200mV"=33, "x10_Probe_500mV"=34, "x10_Probe_1V"=35, "x10_Probe_2V"=36, "x10_Probe_5V"=37, "x10_Probe_10V"=38, "x10_Probe_20V"=39, "x10_Probe_50V"=40, "x10_Probe_100V"=41, "x10_Probe_200V"=42, "x10_Probe_500V"=43, "CURRENT_CLAMP_60A_2A"=10500, "CURRENT_CLAMP_60A_5A"=10501, "CURRENT_CLAMP_60A_10A"=10502, "CURRENT_CLAMP_60A_20A"=10503, "CURRENT_CLAMP_60A_50A"=10504, "CURRENT_CLAMP_60A_60A"=10505, "CURRENT_CLAMP_60A_V2_0_5A"=10600, "CURRENT_CLAMP_60A_V2_1A"=10601, "CURRENT_CLAMP_60A_V2_2A"=10602, "CURRENT_CLAMP_60A_V2_5A"=10603, "CURRENT_CLAMP_60A_V2_10A"=10604, "CURRENT_CLAMP_60A_V2_20A"=10605, "CURRENT_CLAMP_60A_V2_50A"=10606, "CURRENT_CLAMP_60A_V2_60A"=10607, "RESISTANCE_LEAD_NEG5_TO_20OHM"=7000, "RESISTANCE_LEAD_NEG50_TO_200OHM"=7001, "RESISTANCE_LEAD_NEG500_TO_2KOHM"=7002, "RESISTANCE_LEAD_NEG5K_TO_20KOHM"=7003, "RESISTANCE_LEAD_NEG50K_TO_LEAD_200KOHM"=7004, "RESISTANCE_LEAD_NEG500K_TO_LEAD_2MOHM"=7005, "RESISTANCE_LEAD_DIODE_TEST"=7006, "HT_NEG3_TO_5KV"=8950, "HT_NEG3_TO_10KV"=8951, "HT_NEG5_TO_20KV"=8952, "HT_NEG5_TO_50KV"=8953, "HT_NEG5_TO_100KV"=8954, "HT_NEG3_TO_5KV_INVERTED"=8955, "HT_NEG3_TO_10KV_INVERTED"=8956, "HT_NEG5_TO_20KV_INVERTED"=8957, "HT_NEG5_TO_50KV_INVERTED"=8958, "HT_NEG5_TO_100KV_INVERTED"=8959, "TEMPERATURE_NEG50_TO_150DEGC"=9000, "PRESSURE_SENSOR_-100k-150k_PASCALS"=9100, "PRESSURE_SENSOR_-100k_TO_400k_PASCALS"=9101, "PRESSURE_SENSOR_-200k_TO_800k_PASCALS"=9102, "PRESSURE_SENSOR_-400k_TO_1600k_PASCALS"=9103, "PRESSURE_SENSOR_-400k_TO_3400k_PASCALS"=9104, "PRESSURE_SENSOR_-150k_TO_1350k_PASCALS"=9105, "PICO_CONNECT_PROBE_OFF"=1024] ("temp")
                # "Probe Disabled"
              }
              frame True {
                # "Use user 'Range' control if within probe limits"
                n18 = case shown="False" w85 {
                  tunnel: [w86 w87] -> w82
                  tunnel: w83 -> [_ w87]
                  tunnel: w84 -> [w86 _]
                  frame False {
                  }
                  frame True {
                  }
                }
              }
            }
          }
        }
        n19 = To Unsigned Long Integer(number=w46) -> (unsigned 32bit integer=w49:u32)
        n20 = Bundle By Name(cluster=T1 {"Enabled"=FALSE, "Coupling"=1, "Range"=6, "Analogue Offset"=0.0, "Bandwidth Limit"=0} ("Channel A Settings"), "Enabled"=w31, "Coupling"=w57, "Range"=w49, "Analogue Offset"=w56, "Bandwidth Limit"=w30) -> (w44:T1)
        n21 = Bundle By Name(cluster=T6 {"Ch Min Limit"=0.0, "Ch Max Limit"=20000.0, "Probe Name"=0} ("Probe Info"), "Probe Name"=w33, "Ch Min Limit"=w43, "Ch Max Limit"=w42) -> (w45:T6)
        n22 = Bundle("Probe Info"=w45, "Channel A Settings"=w44) -> (w35:T2)  [unwired: 1 in]
      }
      n23 = Index Array(array=w17, index=0) -> (element=→"ChA":T2)
      n24 = Index Array(array=w17, index=1) -> (element=→"ChB":T2)
      n25 = Index Array(array=w17, index=2) -> (element=→"ChC":T2)
      n26 = Index Array(array=w17, index=3) -> (element=→"ChD":T2)
    }
    frame Error {
    }
  }
  "error out" <- w9
  "handle out" <- w10
